vi "Create.vi"(9 "Alias":string, 10 "Queue Actor":refnum<class "Queue Actor.lvclass">, 11 "jettl Queue Actor in":refnum<class "jettl Queue Actor.lvclass">) -> (3 "jettl Queue Actor out":refnum<class "jettl Queue Actor.lvclass">)   [LabVIEW 2021, in "jettl.lvlib" / "jettl Queue Actor.lvlib" / "jettl Queue Actor.lvclass"]
uses:
  jettl Queue Actor.lvclass
  C:/git/jettl/src/Actor/Queue Actor/Queue Actor.lvclass
  Actor/Queue Actor/Queue Actor.lvclass
  State/Nominal State/Nominal State.lvclass
  C:/git/jettl/src/jettl/jettl Queue Actor/State/State/State.lvclass
  jettl Queue Actor.lvclass/jettl Queue Actor.ctl
  Actor/Queue Actor/Loop.vi
  jettl.lvlib
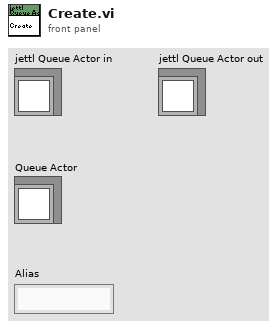
[diagram p1: front panel]
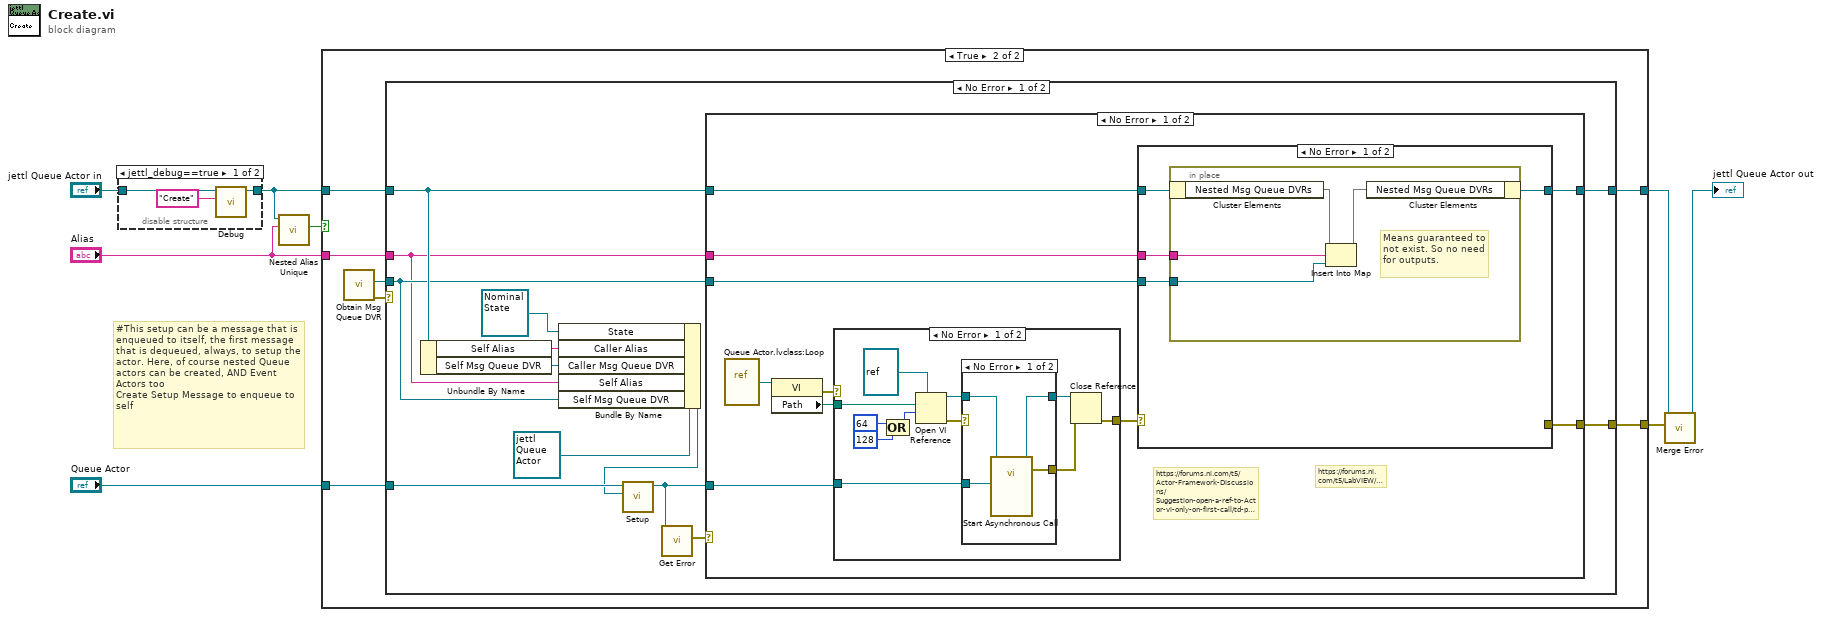
[diagram p0: block diagram]
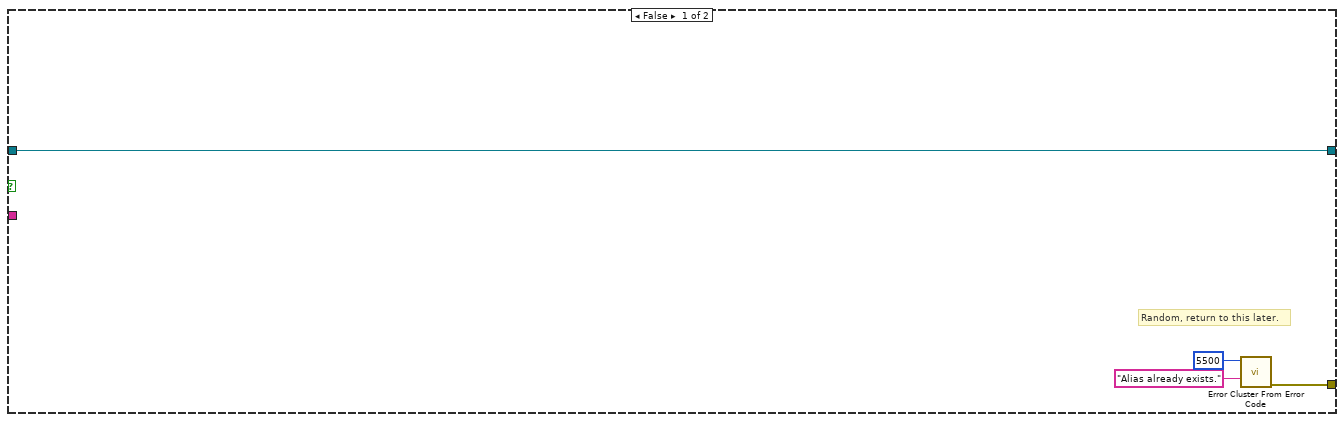
[diagram p2: hidden frame]
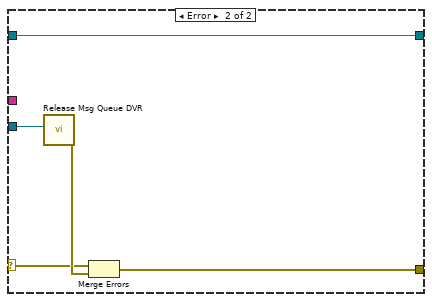
[diagram p5: hidden frame]
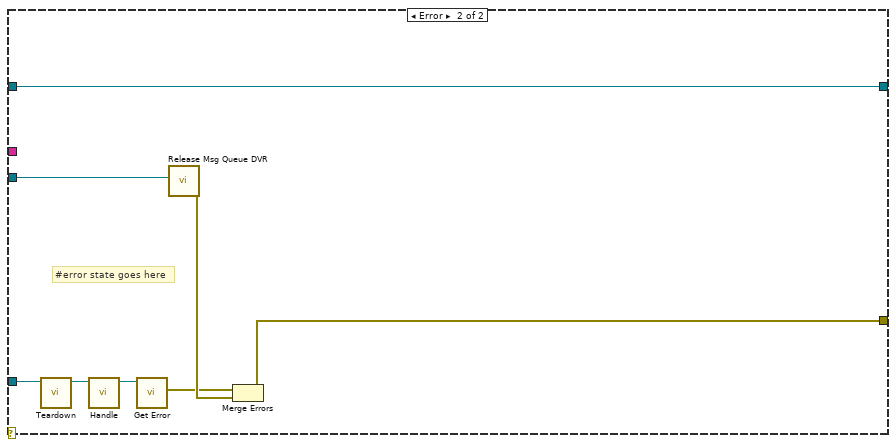
[diagram p6: hidden frame]
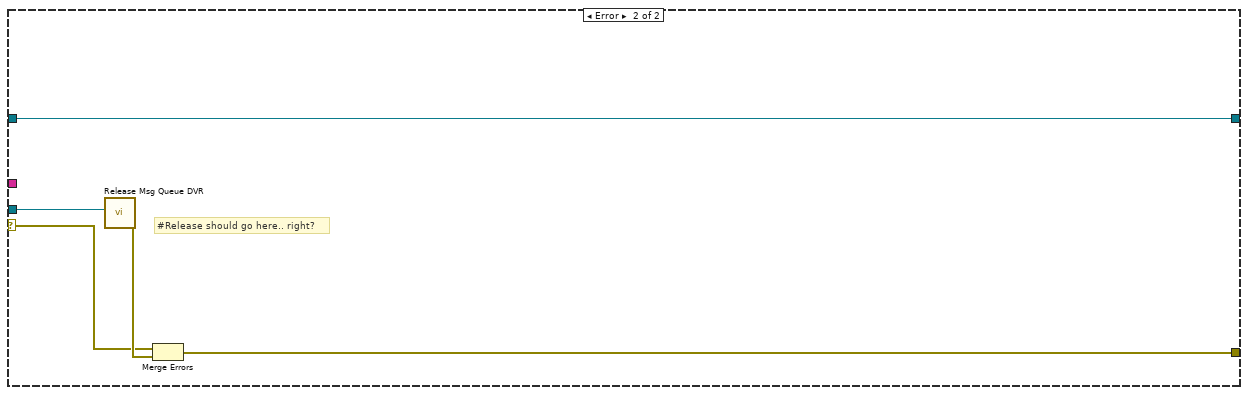
[diagram p7: hidden frame]
diagram:
  # "#This setup can be a message that is enqueued to itself, the first message that is dequeued, always, to setup the actor. Here, of course nested Queue actors can be created, AND Event Actors too\nCreate Setup Message to enqueue to self"
  n1 = disable-structure shown="jettl_debug==true" {
    disable-tunnel: "jettl Queue Actor in" -> [w11 w12]
    disable-tunnel: [w10 w12] -> w6
    frame condition #0 (active) {
      n2 = call "Debug.vi"("Method"="Create", "jettl Queue Actor in"=w11) -> ("jettl Queue Actor out"=w10:refnum<class "jettl Queue Actor.lvclass">)  [unwired: 9 in]
    }
    frame condition #1 {
    }
  }
  n3 = call-dynamic "Nested Alias Unique.vi"("Nested Alias"="Alias", "jettl Queue Actor in"=w6) -> ("Nested Alias Unique?"=w4:bool)  [unwired: 9 in]
  n4 = case shown="True" w4 {
    tunnel: "Queue Actor" -> [_ w23]
    tunnel: [w16 w18] -> w2
    tunnel: w6 -> [w16 w20]
    tunnel: "Alias" -> [_ w17]
    tunnel: [w15 w19] -> w3
    frame False {
      # "Random, return to this later."
      n5 = call <vilib>:"Error Cluster From Error Code.vi"("error message (\"\")"="Alias already exists." ("error message (\"\")"), "error code (0)"=5500) -> ("error out"=w15:errorcluster)  [unwired: 7 in]
    }
    frame True {
      n6 = call "Obtain Msg Queue DVR.vi"() -> ("error out"=w21:errorcluster, "Msg Queue DVR"=w22:refnum<data-value>)  [unwired: 10 in]
      n7 = case shown="No Error" w21 {
        selector: w21 -> [_ w86]
        tunnel: [w36 w90] -> w18
        tunnel: [w35 w88] -> w19
        tunnel: w23 -> [w33 _]
        tunnel: w22 -> [w26 w89]
        tunnel: w20 -> [w32 w90]
        tunnel: w17 -> [w24 _]
        frame No Error {
          n8 = Unbundle By Name(w32) -> ("Self Alias"=w27:string, "Self Msg Queue DVR"=w31:refnum<data-value>)
          n9 = Bundle By Name(cluster=refnum<class "jettl Queue Actor.lvclass"> refnum ("Self Actor in"), "State"=refnum<class "Nominal State.lvclass"> refnum ("LVCAM.lvlib:Msging Self Actor State.lvclass"), "Caller Alias"=w27, "Caller Msg Queue DVR"=w31, "Self Alias"=w24, "Self Msg Queue DVR"=w26) -> (w30:refnum<class "jettl Queue Actor.lvclass">)
          n10 = call-dynamic "Setup.vi"("Queue Actor"=w30, "Queue Actor in"=w33) -> ("Queue Actor out"=w28:refnum<class "Queue Actor.lvclass">)  [unwired: 9 in]
          n11 = call-dynamic "Get Error.vi"("Queue Actor in"=w28) -> ("Error"=w29:errorcluster)  [unwired: 10 in]
          n12 = case shown="No Error" w29 {
            tunnel: [w46 w84] -> w36
            tunnel: w28 -> [w45 w82]
            tunnel: [w44 w83] -> w35
            tunnel: w32 -> [w42 w84]
            tunnel: w26 -> [w41 w85]
            tunnel: w24 -> [w37 _]
            frame No Error {
              # "https://forums.ni.com/t5/LabVIEW/Static-VI-Reference/m-p/3334014#M978333"
              # "https://forums.ni.com/t5/Actor-Framework-Discussions/Suggestion-open-a-ref-to-Actor-vi-only-on-first-call/td-p/3451643/page/4"
              n13 = vi-ref "Queue Actor.lvclass:Loop.vi"() -> (w39:refnum<vi>)
              n14 = property class="VI"(reference=w39) -> (error out=w40:errorcluster, "Path"=w38:path)  [unwired: 1 in, 1 out]
              n15 = case shown="No Error" w40 {
                selector: w40 -> [_ w64]
                tunnel: [w55 w64] -> w43
                tunnel: w38 -> [w51 _]
                tunnel: w45 -> [w47 _]
                frame No Error {
                  n16 = Compound Arithmetic op=OR(64 ("options: Multiple Clones,\n  Fire & Forget"), 128 ("options: Multiple Clones,\n  Fire & Forget")) -> (w53:i32)
                  n17 = Open VI Reference(type specifier VI Refnum (for type only)=refnum<vi> refnum, vi path=w51, options=w53) -> (vi reference=w49:refnum<vi>, error out=w50:errorcluster)  [unwired: 3 in]
                  n18 = case shown="No Error" w50 {
                    selector: w50 -> [_ w63]
                    tunnel: [w61 w62] -> w57
                    tunnel: [w60 w63] -> w56
                    tunnel: w49 -> [w59 w62]
                    tunnel: w47 -> [w58 _]
                    frame No Error {
                      n19 = call-by-ref "Start Asynchronous Call"(reference=w59, "Actor in"=w58) -> (reference out=w61:refnum<vi>, error out=w60:errorcluster)  [unwired: 11 in, 1 out]
                    }
                    frame Error {
                    }
                  }
                  n20 = Close Reference(reference=w57, error in (no error)=w56) -> (error out=w55:errorcluster)
                }
                frame Error {
                }
              }
              n21 = case shown="No Error" w43 {
                selector: w43 -> [_ w73]
                tunnel: w42 -> [w68 w77]
                tunnel: [w67 w77] -> w46
                tunnel: w41 -> [w66 w76]
                tunnel: [_ w75] -> w44
                tunnel: w37 -> [w65 _]
                frame No Error {
                  n22 = in-place {
                    in-place-border: w66 -> [w70]
                    in-place-border: w65 -> [w69]
                    # "Means guaranteed to not exist. So no need for outputs."
                    n23 = in-place-cluster #1(w68) -> ("Nested Msg Queue DVRs"=w72:map{string, refnum<data-value>})
                    n24 = Insert Into Map(map in=w72, key=w69, value=w70) -> (map out=w71:map{string, refnum<data-value>})  [unwired: 2 out]
                    n25 = in-place-cluster #1("Nested Msg Queue DVRs"=w71) -> (w67:refnum<class "jettl Queue Actor.lvclass">)
                  }
                }
                frame Error {
                  n26 = call "Release Msg Queue DVR.vi"("Msg Queue DVR"=w76) -> ("error out"=w74:errorcluster)  [unwired: 10 in]
                  n27 = Merge Errors(w73, w74) -> (w75:errorcluster)
                }
              }
            }
            frame Error {
              # "#error state goes here"
              n28 = call-dynamic "Teardown.vi"("Teardown in"=w82) -> ("Teardown out"=w81:refnum<class "Queue Actor.lvclass">)  [unwired: 10 in]
              n29 = call-dynamic "Handle.vi"("Queue Actor in"=w81) -> ("Queue Actor out"=w80:refnum<class "Queue Actor.lvclass">)  [unwired: 9 in, 1 out]
              n30 = call-dynamic "Get Error.vi"("Queue Actor in"=w80) -> ("Error"=w78:errorcluster)  [unwired: 10 in]
              n31 = call "Release Msg Queue DVR.vi"("Msg Queue DVR"=w85) -> ("error out"=w79:errorcluster)  [unwired: 10 in]
              n32 = Merge Errors(w78, w79) -> (w83:errorcluster)
            }
          }
        }
        frame Error {
          # "#Release should go here.. right?"
          n33 = call "Release Msg Queue DVR.vi"("Msg Queue DVR"=w89) -> ("error out"=w87:errorcluster)  [unwired: 10 in]
          n34 = Merge Errors(w86, w87) -> (w88:errorcluster)
        }
      }
    }
  }
  n35 = call-dynamic "Merge Error.vi"("Error"=w3, "jettl Queue Actor in"=w2) -> ("jettl Queue Actor out"=→"jettl Queue Actor out":refnum<class "jettl Queue Actor.lvclass">)  [unwired: 9 in]
